vi "golpi_struct_test2.vi"() -> ()   [LabVIEW 2013, in "GOLPI library.lvlib"]
uses:
  GOLPI library.lvlib
panel:
  out "Numeric":dbl
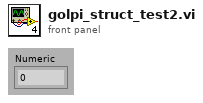
[diagram p1: front panel]
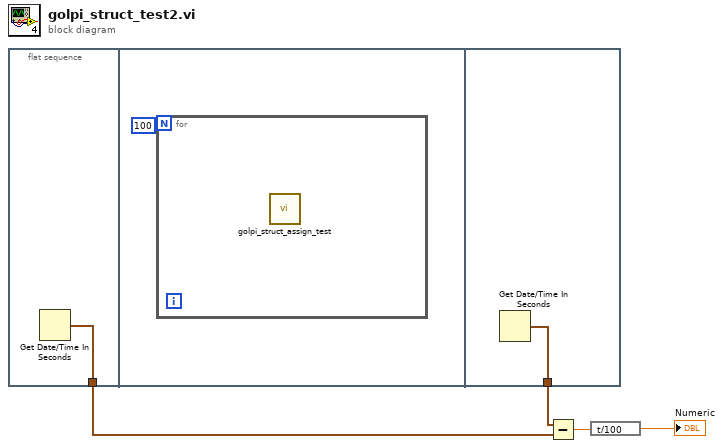
[diagram p0: block diagram]
diagram:
  n1 = flat-sequence {
    tunnel: [w5] -> w3
    tunnel: [w7] -> w4
    frame #0 {
      n2 = Get Date/Time In Seconds() -> (seconds since 1Jan1904=w5:timestamp)
    }
    frame #1 {
      n3 = for {
        N: 100 -> [_]
        n4 = call "golpi_struct_assign_test.vi"() -> ()  [unwired: 11 in, 1 out]
      }
    }
    frame #2 {
      n5 = Get Date/Time In Seconds() -> (seconds since 1Jan1904=w7:timestamp)
    }
  }
  n6 = Subtract(x=w4, y=w3) -> (x-y=w2:dbl)
  n7 = expression code="t/100"(w2) -> (→"Numeric":dbl)
